vi "createTopic.vi"(8 "error in (no error)":errorcluster, 9 "CommandType":T1, 10 "topic":string, 11 "ProgrammaticInitialization in":refnum<class "ProgrammaticInitialization.lvclass">) -> (0 "error out":errorcluster, 1 "vi name":string, 2 "topicVI":string, 3 "ProgrammaticInitialization out":refnum<class "ProgrammaticInitialization.lvclass">)   [LabVIEW 2016, in "ProgrammaticInitialization.lvclass"]
uses:
  ProgrammaticInitialization.lvclass
  commandType.ctl
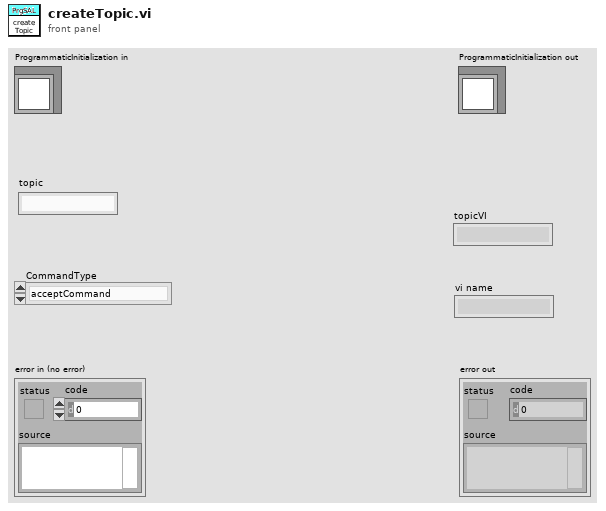
[diagram p1: front panel]
types:
  T1 = typedef "ProgrammaticInitialization.lvclass/commandType.ctl" = enum16{"acceptCommand", "ackCommand", "cancelCallback_command", "cancelCallback_logEvent", "cancelCallback", "flushSamplesEvent", "getEvent", "getNextSample", "getResponse", "getSample", "issueCommand", "logEvent", "monitorCommand", "putSample", "registerCallback_command", "registerCallback_logEvent", "registerCallback", "salCommander", "salEvent", "salProcessor", "salTelemetrySub", "waitForCompletion"}
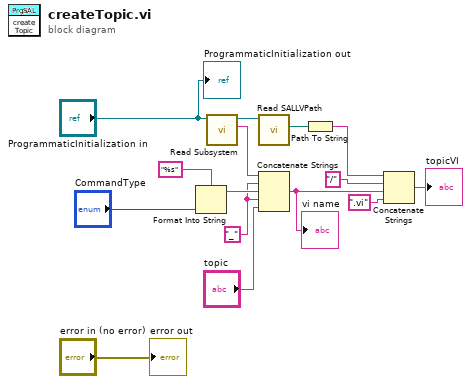
[diagram p0: block diagram]
diagram:
  w4 = "_" ("string")
  n1 = Format Into String(format string="%s", "CommandType") -> (resulting string=w5:string)  [unwired: 2 in, 1 out]
  n2 = call-dynamic "Read Subsystem.vi"("ProgrammaticInitialization in"="ProgrammaticInitialization in") -> ("Subsystem"=w3:string, "ProgrammaticInitialization out"=w10:refnum<class "ProgrammaticInitialization.lvclass">)  [unwired: 8 in, 1 out]
  n3 = call-dynamic "Read SALLVPath.vi"("ProgrammaticInitialization in"=w10) -> ("SALLVPath"=w9:path)  [unwired: 8 in, 2 out]
  n4 = Concatenate Strings(w3, w4, w5, w4, "topic") -> (w2:string)
  "vi name" <- w2
  n5 = Path To String(path=w9) -> (string=w8:string)
  n6 = Concatenate Strings(w8, "/" ("string"), w2, ".vi" ("string")) -> (→"topicVI":string)
  "error out" <- "error in (no error)"
  "ProgrammaticInitialization out" <- "ProgrammaticInitialization in"
